vi "Image in Header or Footer.vi"(0 "report in":refnum<class "NI_Standard Report.lvclass">, 5 "select header or footer":u16(ring) items=["Left Header", "Left Footer", "Center Header", "Center Footer", "Right Herader", "Right Footer"], 9 "image path":string, 11 "error in (no error)":errorcluster, 12 "text above image":string) -> (4 "report out":refnum<class "NI_Standard Report.lvclass">, 15 "error out":errorcluster)   [LabVIEW 2017, in "NI_Standard Report.lvclass"]
doc: "This VI sets an image for the report header or footer.\n\nRemember, with the HTML report type the left, center, and right header texts are placed on separate lines."
uses:
  <vilib>/Utility/NIReport.llb/Standard Report/NI_Standard Report.lvclass
  <vilib>/Utility/NIReport.llb/Standard Report/NI_Standard Report.lvclass/NI_Standard Report.ctl
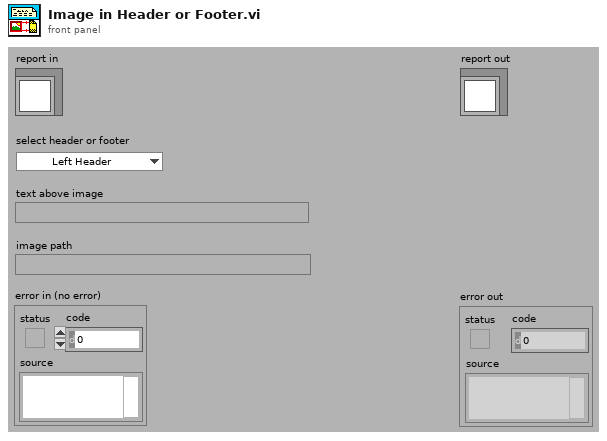
[diagram p1: front panel]
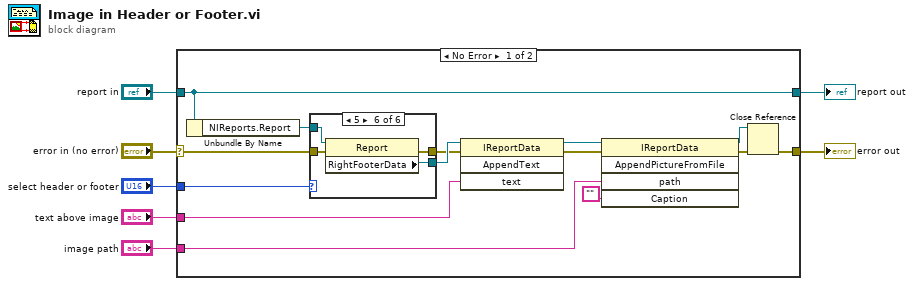
[diagram p0: block diagram]
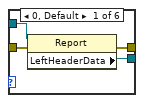
[diagram p2: hidden frame]
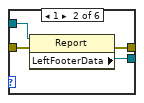
[diagram p3: hidden frame]
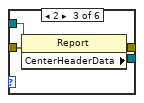
[diagram p4: hidden frame]
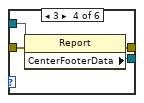
[diagram p5: hidden frame]
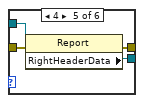
[diagram p6: hidden frame]
diagram:
  n1 = case shown="No Error" "error in (no error)" {
    selector: "error in (no error)" -> [w11 w47]
    tunnel: [w10 w47] -> w6
    tunnel: [w13 w46] -> w4
    tunnel: "report in" -> [w13 w46]
    tunnel: "select header or footer" -> [w12 _]
    tunnel: "text above image" -> [w9 _]
    tunnel: "image path" -> [w8 _]
    frame No Error {
      n2 = Unbundle By Name(w13) -> ("NIReports.Report"=w21:refnum<k7>)
      n3 = case shown="5" w12 {
        tunnel: [w25 w29 w33 w37 w41 w45] -> w18
        tunnel: [w24 w28 w32 w36 w40 w44] -> w17
        tunnel: w11 -> [w23 w27 w31 w35 w39 w43]
        tunnel: w21 -> [w22 w26 w30 w34 w38 w42]
        frame 0, Default {
          n4 = property class="Report"(reference=w22, error in=w23) -> (error out=w24:errorcluster, "LeftHeaderData"=w25:refnum<k7>)  [unwired: 1 out]
        }
        frame 1 {
          n5 = property class="Report"(reference=w26, error in=w27) -> (error out=w28:errorcluster, "LeftFooterData"=w29:refnum<k7>)  [unwired: 1 out]
        }
        frame 2 {
          n6 = property class="Report"(reference=w30, error in=w31) -> (error out=w32:errorcluster, "CenterHeaderData"=w33:refnum<k7>)  [unwired: 1 out]
        }
        frame 3 {
          n7 = property class="Report"(reference=w34, error in=w35) -> (error out=w36:errorcluster, "CenterFooterData"=w37:refnum<k7>)  [unwired: 1 out]
        }
        frame 4 {
          n8 = property class="Report"(reference=w38, error in=w39) -> (error out=w40:errorcluster, "RightHeaderData"=w41:refnum<k7>)  [unwired: 1 out]
        }
        frame 5 {
          n9 = property class="Report"(reference=w42, error in=w43) -> (error out=w44:errorcluster, "RightFooterData"=w45:refnum<k7>)  [unwired: 1 out]
        }
      }
      n10 = invoke class="IReportData" method="AppendText"(reference=w18, error in=w17, "text"=w9) -> (reference out=w20:refnum<k7>, error out=w19:errorcluster)  [unwired: 1 in, 2 out]
      n11 = invoke class="IReportData" method="AppendPictureFromFile"(reference=w20, error in=w19, "path"=w8, "Caption"="") -> (reference out=w16:refnum<k7>, error out=w15:errorcluster)  [unwired: 1 in, 3 out]
      n12 = Close Reference(reference=w16, error in (no error)=w15) -> (error out=w10:errorcluster)
    }
    frame Error {
    }
  }
  "error out" <- w6
  "report out" <- w4
